vi "waitOnIRQ.vi"(8 "error in (no error)":errorcluster, 10 "Timeout":i32, 11 "IModbus in":refnum<class "IModbus.lvclass">) -> (0 "error out":errorcluster, 1 "TimedOut":bool, 2 "IRQs":i32[](array[numeric]), 3 "IModbus out":refnum<class "IModbus.lvclass">)   [LabVIEW 2016, in "RTModbus.lvlib" / "IModbus.lvclass"]
uses:
  IModbus.lvclass
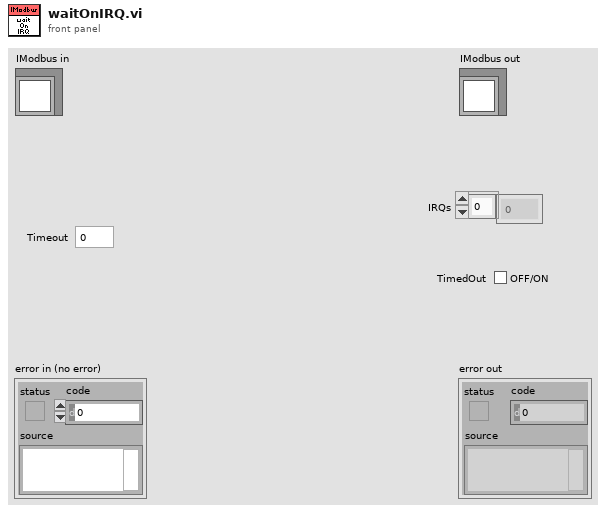
[diagram p1: front panel]
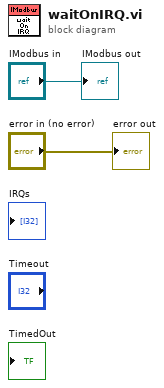
[diagram p0: block diagram]
diagram:
  "error out" <- "error in (no error)"
  "IModbus out" <- "IModbus in"
